vi "calculate_3rdpolynomial_for_height 8.6(subVI).vi"(7 "Total pic. #":i32=45, 8 "Selected \nPeak Location":dbl=7.0, 9 "Z axis height":dbl[](array[numeric]), 10 "Amplitude":dbl[][](array[numeric]), 11 "Peak Location\n(Freq. domain)":dbl[][](array[numeric])) -> (0 "Selected \nPeak Location out":dbl=7.0, 1 "cali-amp.":dbl[](array[numeric]), 2 "Polynomial Coefficients\n(position to amp.)":dbl[](array[numeric]), 3 "Polynomial Coefficients\n(amp. to position)":dbl[](array[numeric]), 4 "Best Polynomial Fit":dbl[](array[numeric]), 6 "cali-stage position":dbl[](array[numeric]))   [LabVIEW 2014]
doc: "This VI fits the selected peak amplitude vs. Z height with 3rd order polynomial."
uses:
  <vilib>/Analysis/NI_AALPro.lvlib
panel:
  in  "stop":bool
  out "residue":dbl
  out "XY Graph":cluster{"Y":dbl[], "Y":dbl[]}[](graph)
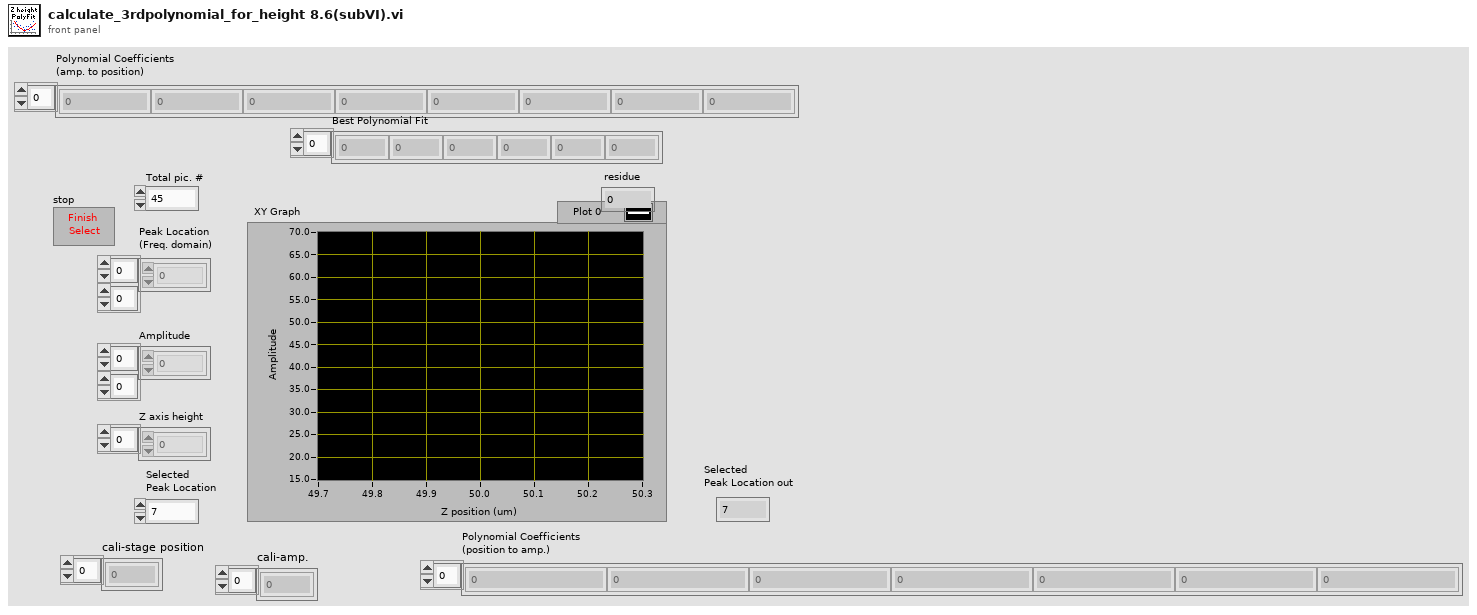
[diagram p1: front panel]
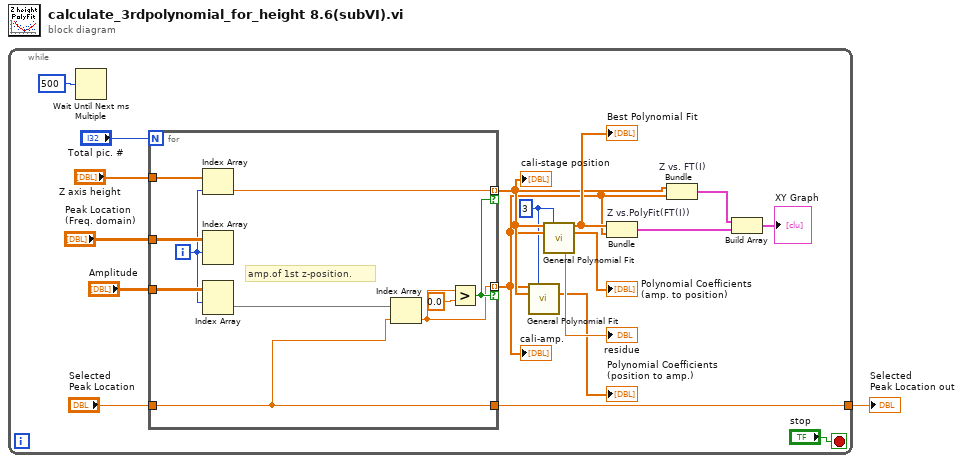
[diagram p0: block diagram]
diagram:
  n1 = while {
    tunnel: [w9] -> w1
    stop <- "stop" stop-if-true
    w2 = 3 ("polynomial order")
    n2 = Wait Until Next ms Multiple(millisecond multiple=u32 500) -> ()  [unwired: 1 out]
    n3 = for {
      N: "Total pic. #" -> [_]
      tunnel: "Peak Location\n(Freq. domain)" -> [w29]
      tunnel: "Selected \nPeak Location" -> [w20]
      tunnel: "Amplitude" -> [w28]
      tunnel: [w21] -> w3 mode=indexing if=w24
      tunnel: "Z axis height" -> [w26]
      tunnel: [w25] -> w7 mode=indexing if=w24
      tunnel: [w20] -> w9
      i -> [w23]
      # "amp.of 1st z-position."
      n4 = Index Array(array=w26, index=w23) -> (element=w25:dbl)
      n5 = Index Array(array=w29, index (row)=w23) -> ()  [unwired: 1 in, 1 out]
      n6 = Index Array(array=w28, index (row)=w23) -> (element=w22:dbl[])  [unwired: 1 in]
      n7 = Index Array(array=w22, index=w20) -> (element=w21:dbl)
      n8 = Greater?(x=w21, y=0.0) -> (0:w24:bool)
    }
    "cali-stage position" <- w7
    "cali-amp." <- w3
    n9 = call <vilib>:"General Polynomial Fit.vi"("Y"=w3, "polynomial order"=w2, "X"=w7) -> ("Polynomial Coefficients"=→"Polynomial Coefficients\n(position to amp.)":dbl[])  [unwired: 9 in, 3 out]
    n10 = call <vilib>:"General Polynomial Fit.vi"("Y"=w7, "polynomial order"=w2, "X"=w3) -> ("Best Polynomial Fit"=w8:dbl[], "Polynomial Coefficients"=→"Polynomial Coefficients\n(amp. to position)":dbl[], "residue"=→"residue":dbl)  [unwired: 9 in, 1 out]
    "Best Polynomial Fit" <- w8
    n11 = Bundle "Z vs.PolyFit(FT(I))"("Best Polynomial Fit"=w8, w3) -> (w16:cluster{"Best Polynomial Fit":dbl[], dbl[]})  [unwired: 1 out]
    n12 = Bundle "Z vs. FT(I)"(w7, w3) -> (w17:cluster{dbl[], dbl[]})  [unwired: 1 out]
    n13 = Build Array(w17, w16) -> (→"XY Graph":cluster{"Best Polynomial Fit":dbl[], dbl[]}[])
  }
  "Selected \nPeak Location out" <- w1
